vi "Angle From Pixel.vi"(10 "Pixel":dbl, 11 "Angle Aperture":dbl) -> (3 "Theta":dbl)   [LabVIEW 2016]
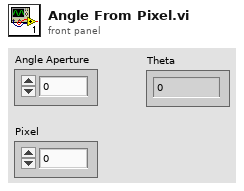
[diagram p1: front panel]
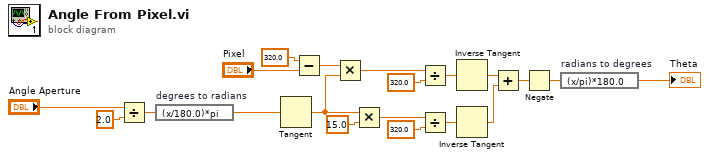
[diagram p0: block diagram]
diagram:
  n1 = Divide(x="Angle Aperture", y=2.0) -> (x/y=w3:dbl)
  n2 = expression code="(x/180.0)*pi" "degrees to radians"(w3) -> (w2:dbl)
  n3 = Tangent(1:w2) -> (0:w13:dbl)
  n4 = Subtract(x=320.0, y="Pixel") -> (x-y=w4:dbl)
  n5 = Multiply(x=w4, y=w13) -> (x*y=w16:dbl)
  n6 = Multiply(x=w13, y=15.0) -> (x*y=w11:dbl)
  n7 = Divide(x=w16, y=320.0) -> (x/y=w17:dbl)
  n8 = Divide(x=w11, y=320.0) -> (x/y=w9:dbl)
  n9 = Inverse Tangent(1:w17) -> (0:w8:dbl)
  n10 = Inverse Tangent(1:w9) -> (0:w7:dbl)
  n11 = Add(x=w8, y=w7) -> (x+y=w6:dbl)
  n12 = Negate(x=w6) -> (-x=w1:dbl)
  n13 = expression code="(x/pi)*180.0" "radians to degrees"(w1) -> (→"Theta":dbl)
